vi "Wavelength Digikröm.vi"(8 "error in (no error)":errorcluster, 10 "Spectrometer Digikröm.lvclass":refnum<class "Spectrometer Digikröm.lvclass">, 11 "Wavelength Digikröm in":refnum<class "Wavelength Digikröm.lvclass">) -> (0 "error out":errorcluster, 3 "Wavelength Digikröm out":refnum<class "Wavelength Digikröm.lvclass">)   [LabVIEW 2009, in "Wavelength Digikröm.lvclass"]
uses:
  Wavelength Digikröm.lvclass
  Instruments/Spectrometer Digikröm/Spectrometer Digikröm.lvclass
  Scanner/Scanner.lvclass
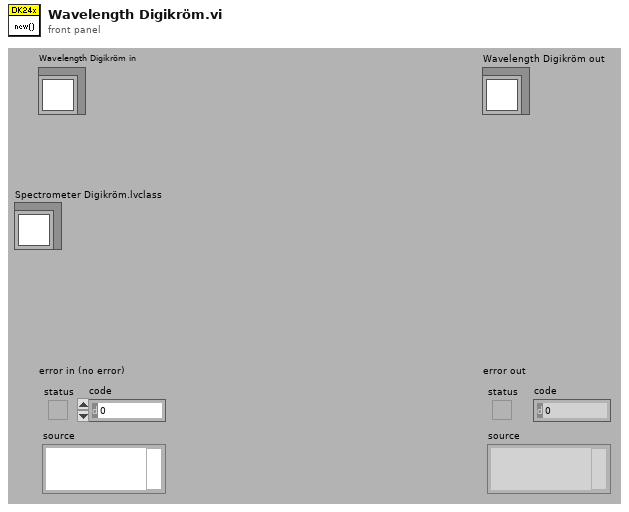
[diagram p1: front panel]
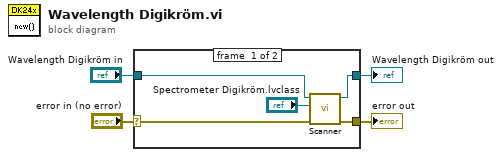
[diagram p0: block diagram]
diagram:
  n1 = case shown="No Error" "error in (no error)" {
    selector: "error in (no error)" -> [w7 w11]
    tunnel: [w6 w11] -> w3
    tunnel: [w8 w10] -> w1
    tunnel: "Wavelength Digikröm in" -> [w9 w10]
    frame #0 {
      n2 = call "Scanner.vi"("error in (no error)"=w7, "Scannable"="Spectrometer Digikröm.lvclass", "Scanner.lvclass in"=w9) -> ("error out"=w6:errorcluster, "Scanner.lvclass out"=w8:refnum<class "Wavelength Digikröm.lvclass">)  [unwired: 1 in, 6 out]
    }
    frame #1 {
    }
  }
  "error out" <- w3
  "Wavelength Digikröm out" <- w1
